vi "GetPosition.vi"(8 "error in (no error)":errorcluster, 11 "DirectedGraphMapNode in":refnum<class "NI_Robotics_DirectedGraphMapNode.lvclass">) -> (0 "error out":errorcluster, 1 "coordinates":dbl[](array[numeric]), 2 "name":string, 3 "DirectedGraphMapNode out":refnum<class "NI_Robotics_DirectedGraphMapNode.lvclass">)   [LabVIEW 2017, in "NI_Robotics_DirectedGraphMapNode.lvclass"]
uses:
  <vilib>/robotics/Navigation/shared/MapNode/DirectedGraphMapNode/NI_Robotics_DirectedGraphMapNode.lvclass
  <vilib>/robotics/Navigation/shared/MapNode/DirectedGraphMapNode/NI_Robotics_DirectedGraphMapNode.lvclass/NI_Robotics_DirectedGraphMapNode.ctl
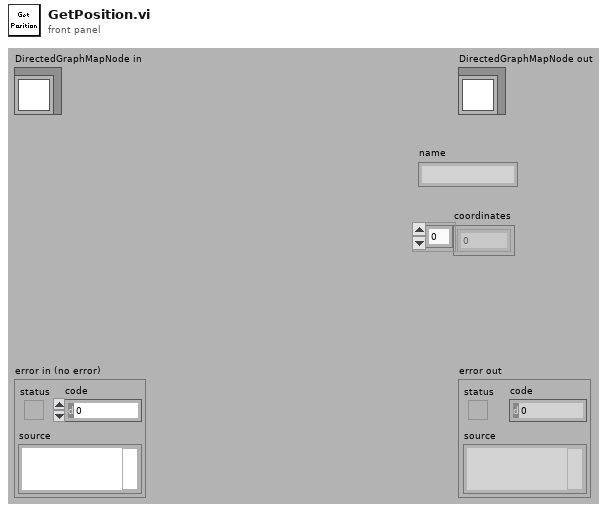
[diagram p1: front panel]
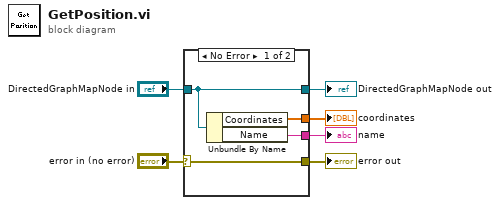
[diagram p0: block diagram]
diagram:
  n1 = case shown="No Error" "error in (no error)" {
    selector: "error in (no error)" -> [w10 w12]
    tunnel: [w10 w12] -> w5
    tunnel: [w9 w11] -> w3
    tunnel: "DirectedGraphMapNode in" -> [w9 w11]
    tunnel: [w8 _] -> w2
    tunnel: [w7 _] -> w1
    frame No Error {
      n2 = Unbundle By Name(w9) -> ("Coordinates"=w8:dbl[], "Name"=w7:string)
    }
    frame Error {
    }
  }
  "error out" <- w5
  "DirectedGraphMapNode out" <- w3
  "coordinates" <- w2
  "name" <- w1
